vi "GPSGetDate.vi"(0 "error in (no error)":errorcluster, 3 "Device In":u64) -> (7 "error out":errorcluster, 9 "Date":T1, 10 "Device Out":u64)   [LabVIEW 2012, in "Phidget GPS.lvlib"]
doc: "${Date:Header}"
uses:
  <instrlib>/Phidgets/Phidget GPS/Phidget GPS.lvlib
  <instrlib>/Phidgets/Phidget Common/Phidget Common.lvlib
  phidget22.dll
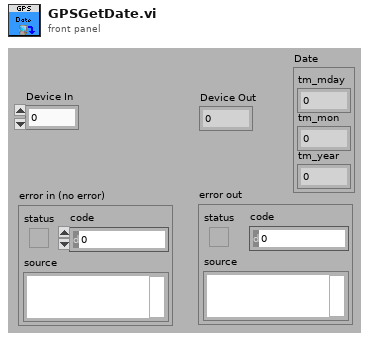
[diagram p1: front panel]
types:
  T1 = cluster{"tm_mday":i16, "tm_mon":i16, "tm_year":i16}
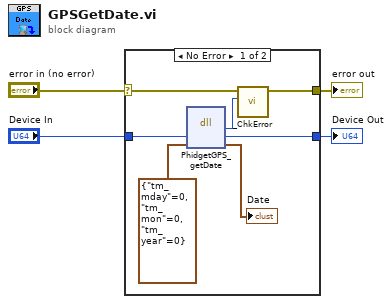
[diagram p0: block diagram]
diagram:
  n1 = case shown="No Error" "error in (no error)" {
    selector: "error in (no error)" -> [w8 w13]
    tunnel: [w7 w13] -> w3
    tunnel: "Device In" -> [w11 w12]
    tunnel: [w10 w12] -> w1
    frame No Error {
      n2 = dll-call lib="phidget22.*" fn="PhidgetGPS_getDate" ("phidget21.*:CPhidgetGPS_getDate")("phid"=w11, "Data"=T1 {"tm_mday"=0, "tm_mon"=0, "tm_year"=0}) -> ("return type"=w9:i32, "phid"=w10:u64, "Data"=→"Date":T1)  [unwired: 3 in, 2 out]
      n3 = call <instrlib>:"_ChkError.vi"("Return Code"=w9, "error in (no error)"=w8) -> ("error out"=w7:errorcluster)  [unwired: 9 in]
    }
    frame Error {
    }
  }
  "error out" <- w3
  "Device Out" <- w1
